vi "PicoLog1000ExampleBlock.vi"() -> ()   [LabVIEW 2010]
panel:
  out "UnitInfo":T1
  out "Sample Interval (s)":dbl=4e-06 format="%#_4p"
  out "Waveform Graph":cluster{i32, dbl, dbl[][]}(graph)={0, 4e-06, []}
  in  "Trigger":T2={"Enabled"=FALSE, "AutoTrigger"=FALSE, "Delay (%)"=-50.0, "Auto Trigger\nTiime (ms)"=1000, "Channel"=1, "Trigger Direction"=0, "threshold (mV)"=500, "hysteresis (mV)"=5} {"Trigger Direction" items=["rising edge", "falling edge"]; "Channel" items=["Ch1"=1, "Ch2"=2, "Ch3"=3, "Ch4"=4, "Ch5"=5, "Ch6"=6, "Ch7"=7, "Ch8"=8, "Ch9"=9, "Ch10"=10, "Ch11"=11, "Ch12"=12, "Ch13"=13, "Ch14"=14, "Ch15"=15, "Ch16"=16]}
  out "Triggered":bool
  out "noOfValues collected per ch":u32=1000
  in  "Number of sample per channel":u32=1000
  in  "Block length (us)":u32=1000
  in  "Channels Enabled":string="1,2,3,4" caption="Channels Enabled (1,2,3)"
  in  "stop":bool
  out "Ch Over Range":bool[](array[boolean])
  out "Ready":bool
  out "pl1000 handle out":i16=16384
  out "error out":errorcluster
  in  "error in (no error)":errorcluster
  # "Block Mode Example"
  # "This example sets the trigger, collects a single block of data and\ndisplays it"
  # "Trigger delay of \n-50% means the\ntrigger event is\nin the middle of \nthe block"
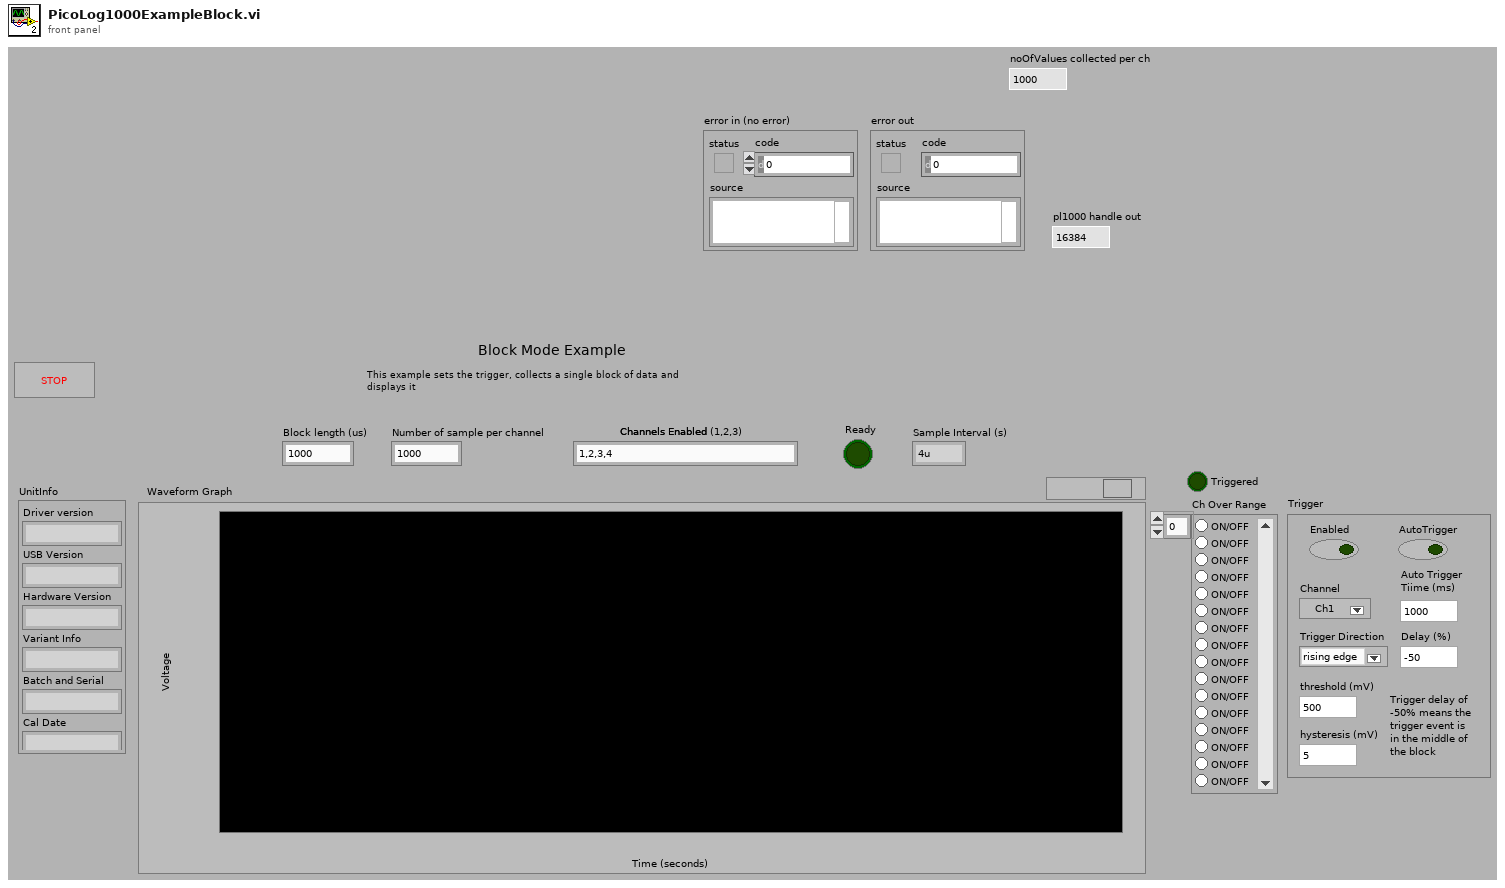
[diagram p1: front panel]
types:
  T1 = cluster{"Driver version":string, "USB Version":string, "Hardware Version":string, "Variant Info":string, "Batch and Serial":string, "Cal Date":string, "[6]":string, "[7]":string, "[8]":string}
  T2 = cluster{"Enabled":bool, "AutoTrigger":bool, "Delay (%)":sgl, "Auto Trigger\nTiime (ms)":u16, "Channel":u16, "Trigger Direction":u16, "threshold (mV)":u16, "hysteresis (mV)":u16}
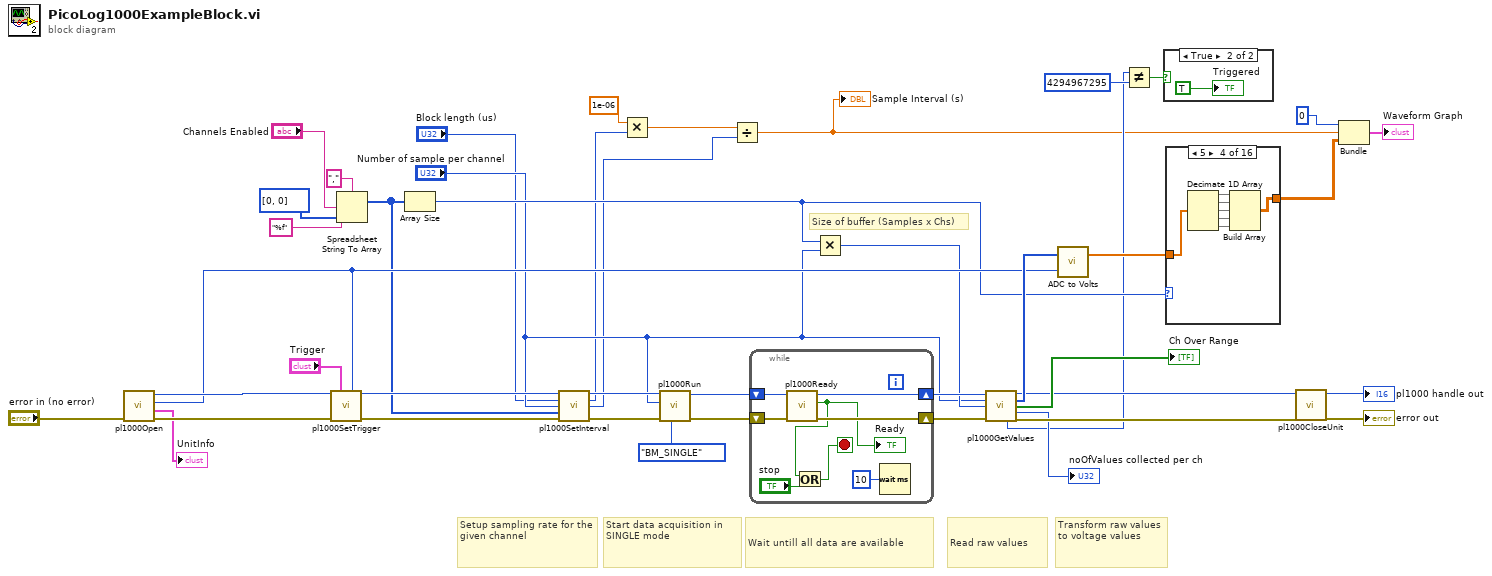
[diagram p0: block diagram]
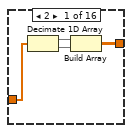
[diagram p3: hidden frame]
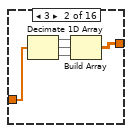
[diagram p4: hidden frame]
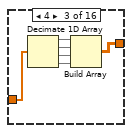
[diagram p5: hidden frame]
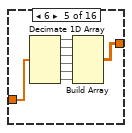
[diagram p6: hidden frame]
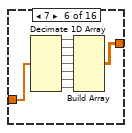
[diagram p7: hidden frame]
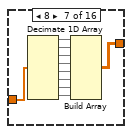
[diagram p8: hidden frame]
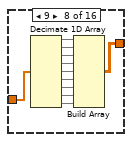
[diagram p9: hidden frame]
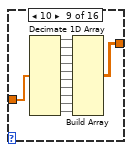
[diagram p10: hidden frame]
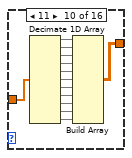
[diagram p11: hidden frame]
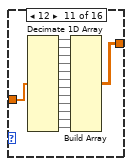
[diagram p12: hidden frame]
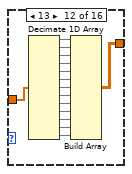
[diagram p13: hidden frame]
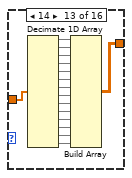
[diagram p14: hidden frame]
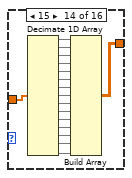
[diagram p15: hidden frame]
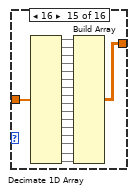
[diagram p16: hidden frame]
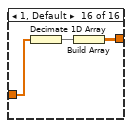
[diagram p17: hidden frame]
diagram:
  # "Size of buffer (Samples x Chs)"
  # "Transform raw values to voltage values"
  # "Read raw values"
  # "Wait untill all data are available"
  # "Start data acquisition in SINGLE mode"
  # "Setup sampling rate for the given channel"
  n1 = call "pl1000Open.vi"("error in (no error)"="error in (no error)") -> ("error out"=w29:errorcluster, "UnitInfo"=→"UnitInfo":T1, "maxValue"=w25:u16, "pl1000 handle out"=w28:i16)  [unwired: 7 in]
  n2 = call "pl1000SetTrigger.vi"("pl1000 handle"=w28, "Trigger"="Trigger", "maxValue"=w25, "error in (no error)"=w29) -> ("pl1000 handle out"=w26:i16, "error out"=w27:errorcluster)  [unwired: 10 in]
  n3 = Spreadsheet String To Array(delimiter (Tab)=",", format string="%f", spreadsheet string="Channels Enabled", array type (2D Dbl)=u32[] [0, 0]) -> (array=w20:u32[])
  n4 = Array Size(array=w20) -> (size(s)=w16:i32)
  n5 = call "pl1000SetInterval.vi"("pl1000 handle"=w26, "usForBlock"="Block length (us)", "idealNoOfSamples"="Number of sample per channel", "channels"=w20, "error in (no error)"=w27) -> ("pl1000 handle out"=w37:i16, "usForBlock OP"=w5:u32, "idealNoOfSamples OP"=w3:u32, "error out"=w36:errorcluster)  [unwired: 7 in]
  n6 = Multiply(x=1e-06, y=w5) -> (x*y=w4:dbl)
  n7 = call "pl1000Run.vi"("method"=enum16{"BM_SINGLE", "BM_WINDOW", "BM_STREAM"}."BM_SINGLE", "error in (no error)"=w36, "noOfValues"="Number of sample per channel", "pl1000 handle"=w37) -> ("error out"=w40:errorcluster, "pl1000 handle out"=w41:i16)  [unwired: 6 in]
  n8 = Divide(x=w4, y=w3) -> (x/y=w2:dbl)
  "Sample Interval (s)" <- w2
  n9 = while {
    shift-right: [w49] -> w39
    shift-left: w41 -> [w51]
    shift-right: [w48] -> w38
    shift-left: w40 -> [w50]
    stop <- w45 stop-if-true
    n10 = call "pl1000Ready.vi"("error in (no error)"=w50, "pl1000 handle"=w51) -> ("error out"=w48:errorcluster, "ready"=w44:bool, "pl1000 handle out"=w49:i16)  [unwired: 7 in]
    "Ready" <- w44
    n11 = Or(x=w44, y="stop") -> (x .or. y?=w45:bool)
    n12 = Wait (ms)(milliseconds to wait=u32 10) -> ()  [unwired: 1 out]
  }
  n13 = Multiply(x=w16, y="Number of sample per channel") -> (x*y=w17:u32)
  n14 = call "pl1000GetValues.vi"("pl1000 handle"=w39, "noOfValues"="Number of sample per channel", "SizeOfArray"=w17, "error in (no error)"=w38) -> ("pl1000 handle out"=w32:i16, "values"=w35:u16[], "Ch Over Range"=→"Ch Over Range":bool[], "noOfValues collected per ch"=→"noOfValues collected per ch":u32, "triggerIndex"=w12:u32, "error out"=w33:errorcluster)  [unwired: 6 in]
  n15 = call "ADC to Volts.vi"("maxValue"=w25, "ADC values"=w35) -> ("values in Volt"=w19:dbl[])  [unwired: 1 in]
  n16 = Not Equal?(x=w12, y=u32 4294967295) -> (x != y?=w14:bool)
  n17 = case shown="True" w14 {
    frame False {
    }
    frame True {
      "Triggered" <- TRUE ("Boolean")
    }
  }
  n18 = case shown="5" w16 {
    tunnel: [w54 w59 w65 w72 w80 w89 w99 w110 w122 w135 w149 w164 w180 w197 w215 w219] -> w9
    tunnel: w19 -> [w53 w57 w62 w68 w75 w83 w92 w102 w113 w125 w138 w152 w167 w183 w200 w218]
    frame 2 {
      n19 = Decimate 1D Array(w53) -> (w56:dbl[], w55:dbl[])
      n20 = Build Array(w56, w55) -> (w54:dbl[][])
    }
    frame 3 {
      n21 = Decimate 1D Array(w57) -> (w61:dbl[], w60:dbl[], w58:dbl[])
      n22 = Build Array(w61, w60, w58) -> (w59:dbl[][])
    }
    frame 4 {
      n23 = Decimate 1D Array(w62) -> (w67:dbl[], w66:dbl[], w64:dbl[], w63:dbl[])
      n24 = Build Array(w67, w66, w64, w63) -> (w65:dbl[][])
    }
    frame 5 {
      n25 = Decimate 1D Array(w68) -> (w74:dbl[], w73:dbl[], w71:dbl[], w70:dbl[], w69:dbl[])
      n26 = Build Array(w74, w73, w71, w70, w69) -> (w72:dbl[][])
    }
    frame 6 {
      n27 = Decimate 1D Array(w75) -> (w82:dbl[], w81:dbl[], w79:dbl[], w78:dbl[], w77:dbl[], w76:dbl[])
      n28 = Build Array(w82, w81, w79, w78, w77, w76) -> (w80:dbl[][])
    }
    frame 7 {
      n29 = Decimate 1D Array(w83) -> (w91:dbl[], w90:dbl[], w88:dbl[], w87:dbl[], w86:dbl[], w85:dbl[], w84:dbl[])
      n30 = Build Array(w91, w90, w88, w87, w86, w85, w84) -> (w89:dbl[][])
    }
    frame 8 {
      n31 = Decimate 1D Array(w92) -> (w101:dbl[], w100:dbl[], w98:dbl[], w97:dbl[], w96:dbl[], w95:dbl[], w94:dbl[], w93:dbl[])
      n32 = Build Array(w101, w100, w98, w97, w96, w95, w94, w93) -> (w99:dbl[][])
    }
    frame 9 {
      n33 = Decimate 1D Array(w102) -> (w112:dbl[], w111:dbl[], w109:dbl[], w108:dbl[], w107:dbl[], w106:dbl[], w105:dbl[], w104:dbl[], w103:dbl[])
      n34 = Build Array(w112, w111, w109, w108, w107, w106, w105, w104, w103) -> (w110:dbl[][])
    }
    frame 10 {
      n35 = Decimate 1D Array(w113) -> (w124:dbl[], w123:dbl[], w121:dbl[], w120:dbl[], w119:dbl[], w118:dbl[], w117:dbl[], w116:dbl[], w115:dbl[], w114:dbl[])
      n36 = Build Array(w124, w123, w121, w120, w119, w118, w117, w116, w115, w114) -> (w122:dbl[][])
    }
    frame 11 {
      n37 = Decimate 1D Array(w125) -> (w137:dbl[], w136:dbl[], w134:dbl[], w133:dbl[], w132:dbl[], w131:dbl[], w130:dbl[], w129:dbl[], w128:dbl[], w127:dbl[], w126:dbl[])
      n38 = Build Array(w137, w136, w134, w133, w132, w131, w130, w129, w128, w127, w126) -> (w135:dbl[][])
    }
    frame 12 {
      n39 = Decimate 1D Array(w138) -> (w151:dbl[], w150:dbl[], w148:dbl[], w147:dbl[], w146:dbl[], w145:dbl[], w144:dbl[], w143:dbl[], w142:dbl[], w141:dbl[], w140:dbl[], w139:dbl[])
      n40 = Build Array(w151, w150, w148, w147, w146, w145, w144, w143, w142, w141, w140, w139) -> (w149:dbl[][])
    }
    frame 13 {
      n41 = Decimate 1D Array(w152) -> (w166:dbl[], w165:dbl[], w163:dbl[], w162:dbl[], w161:dbl[], w160:dbl[], w159:dbl[], w158:dbl[], w157:dbl[], w156:dbl[], w155:dbl[], w154:dbl[], w153:dbl[])
      n42 = Build Array(w166, w165, w163, w162, w161, w160, w159, w158, w157, w156, w155, w154, w153) -> (w164:dbl[][])
    }
    frame 14 {
      n43 = Decimate 1D Array(w167) -> (w182:dbl[], w181:dbl[], w179:dbl[], w178:dbl[], w177:dbl[], w176:dbl[], w175:dbl[], w174:dbl[], w173:dbl[], w172:dbl[], w171:dbl[], w170:dbl[], w169:dbl[], w168:dbl[])
      n44 = Build Array(w182, w181, w179, w178, w177, w176, w175, w174, w173, w172, w171, w170, w169, w168) -> (w180:dbl[][])
    }
    frame 15 {
      n45 = Decimate 1D Array(w183) -> (w199:dbl[], w198:dbl[], w196:dbl[], w195:dbl[], w194:dbl[], w193:dbl[], w192:dbl[], w191:dbl[], w190:dbl[], w189:dbl[], w188:dbl[], w187:dbl[], w186:dbl[], w185:dbl[], w184:dbl[])
      n46 = Build Array(w199, w198, w196, w195, w194, w193, w192, w191, w190, w189, w188, w187, w186, w185, w184) -> (w197:dbl[][])
    }
    frame 16 {
      n47 = Decimate 1D Array(w200) -> (w217:dbl[], w216:dbl[], w214:dbl[], w213:dbl[], w212:dbl[], w211:dbl[], w210:dbl[], w209:dbl[], w208:dbl[], w207:dbl[], w206:dbl[], w205:dbl[], w204:dbl[], w203:dbl[], w202:dbl[], w201:dbl[])
      n48 = Build Array(w217, w216, w214, w213, w212, w211, w210, w209, w208, w207, w206, w205, w204, w203, w202, w201) -> (w215:dbl[][])
    }
    frame 1, Default {
      n49 = Decimate 1D Array(w218) -> (w220:dbl[])
      n50 = Build Array(w220) -> (w219:dbl[][])
    }
  }
  n51 = call "pl1000CloseUnit.vi"("error in (no error)"=w33, "pl1000 handle"=w32) -> ("error out"=→"error out":errorcluster, "pl1000 handle out"=→"pl1000 handle out":i16)  [unwired: 8 in]
  n52 = Bundle(0, w2, w9) -> (→"Waveform Graph":cluster{i32, dbl, dbl[][]})  [unwired: 1 in]
